vi "Get Value by Array (Numeric).vi"(8 "error in (no error)":errorcluster, 10 "Keys":string[](array[string]), 11 "JSON Object in":refnum<class "JSON Helper.lvclass">) -> (0 "error out":errorcluster, 2 "JSON Numeric out":refnum<class "JSON Numeric.lvclass">)   [LabVIEW 2016]
uses:
  JSON Helper/JSON Helper.lvclass
  JSON Helper/To More Specific Type (Numeric).vi
  JSON Numeric/JSON Numeric.lvclass
  JSON Datatype/JSON Null.lvclass
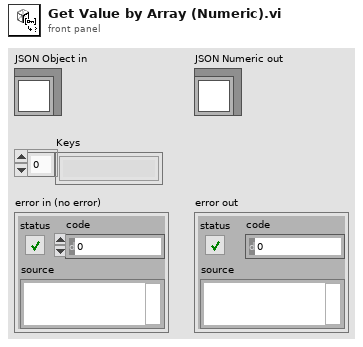
[diagram p1: front panel]
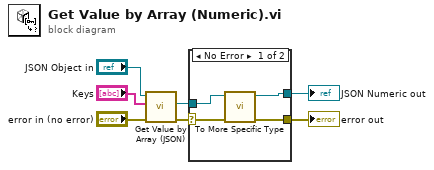
[diagram p0: block diagram]
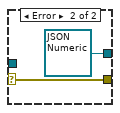
[diagram p2: hidden frame]
diagram:
  n1 = call "Get Value by Array (JSON).vi"("error in (no error)"="error in (no error)", "Keys"="Keys", "JSON in"="JSON Object in") -> ("error out"=w4:errorcluster, "JSON out"=w3:refnum<class "JSON Helper.lvclass">)  [unwired: 7 in]
  n2 = case shown="No Error" w4 {
    selector: w4 -> [w11 w12]
    tunnel: w3 -> [w10 _]
    tunnel: [w9 refnum<class "JSON Numeric.lvclass"> refnum ("JSON Datatype out")] -> w2
    tunnel: [w8 w12] -> w1
    frame No Error {
      n3 = call-poly "To More Specific Type.vi"("error in (no error)"=w11, "JSON Datatype in"=w10) -> ("error out"=w8:errorcluster, "JSON Numeric out"=w9:refnum<class "JSON Numeric.lvclass">)  [unwired: 8 in]
    }
    frame Error {
    }
  }
  "JSON Numeric out" <- w2
  "error out" <- w1
